vi "lightsource-emission-stop.vi"(2 "NKT Input":T2={"Emission"=FALSE, "Operation Mode"=FALSE, "Power Level"=5.0, "Feedback Level"=0.0, "Short Wavelength (nm)"=560, "Long Wavelength (nm)"=580, "UV Wavelength (nm)"=400} {"UV Wavelength (nm)" min=350 max=480 step=1; "Long Wavelength (nm)" min=400 max=850 step=1; "Short Wavelength (nm)" min=400 max=850 step=1; "Feedback Level" min=0.0 max=90.0 step=0.1 format="%.1f%%"; "Power Level" min=5.0 max=100.0 step=0.1 format="%.1f%%"}, 3 "VISA in":refnum<visa-resource-name>) -> (0 "NKT Output":T1 {"Feedback Level" format="%.1f%%"; "Power Level" format="%.1f%%"; "Temp (°C)" format="%.1f"}, 1 "VISA out":refnum<visa-resource-name>)   [LabVIEW 2015]
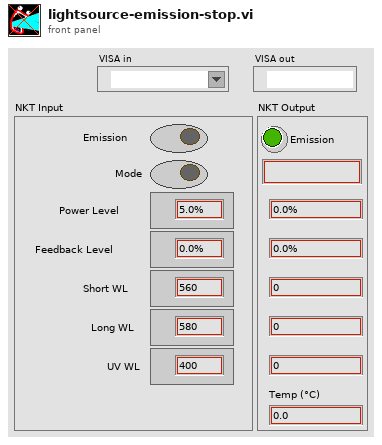
[diagram p1: front panel]
types:
  T1 = cluster{"Emission":bool, "Operation Mode":string, "Power Level":dbl, "Feedback Level":dbl, "Short Wavelength (nm)":i32, "Long Wavelength (nm)":i32, "UV Wavelength (nm)":i32, "Temp (°C)":dbl}
  T2 = cluster{"Emission":bool, "Operation Mode":bool, "Power Level":dbl, "Feedback Level":dbl, "Short Wavelength (nm)":i32, "Long Wavelength (nm)":i32, "UV Wavelength (nm)":i32}
  T3 = cluster{"Emission":bool, "Operation Mode":string, "Power Level":dbl, "Feedback Level":dbl, "Short Wavelength (nm)":dbl, "Long Wavelength (nm)":dbl, "UV Wavelength (nm)":dbl, "Temp (°C)":dbl}
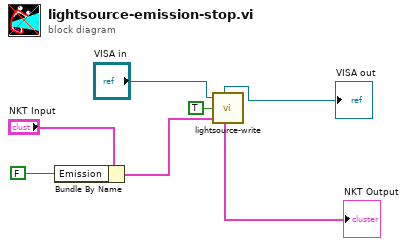
[diagram p0: block diagram]
diagram:
  n1 = Bundle By Name(cluster="NKT Input", "Emission"=FALSE ("Emission On/Off")) -> (w6:T2)
  n2 = call "lightsource-write.vi"("VISA in"="VISA in", "set parameters"=TRUE ("Init NKT?"), "NKT Input"=w6) -> ("VISA out"=→"VISA out":refnum<visa-resource-name>, "NKT Output"=→"NKT Output":T3)  [unwired: 3 in, 1 out]
